vi "test.vi"() -> ()   [LabVIEW 2019]
uses:
  <vilib>/Platform/TimedLoop/XDataNode/timing_clust.ctl
  <vilib>/Platform/TimedLoop/XDataNode/nitl_modes.ctl
  <vilib>/Platform/TimedLoop/XDataNode/wakeup.ctl
  <vilib>/platform/TimedLoop/XDataNode/XDataNode.xnode
  KNRm_ReMi_OS6_436Motor.lvlibp
  <vilib>/Platform/TimedLoop/XDataNode/XDNodeRunTimeDep.lvlib
panel:
  out "Distance (cm)":cluster{"IR1":dbl, "IR2":dbl}
  in  "PulseRate&Dir P/S":dbl format="%#_13g"
  out "PulseCounter+/-":i32
  out "LimitBtn":bool
  in  "stop":bool
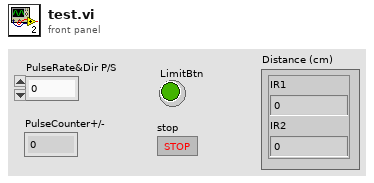
[diagram p1: front panel]
types:
  T1 = typedef "XDNodeRunTimeDep.lvlib/timing_clust.ctl" = cluster{"Expected End [f-1]":u64, "Actual End [f-1]":u64, "Finished Late? [f-1]":bool, "Expected End [i-1]":u64, "Actual End [i-1]":u64, "Finished Late? [i-1]":bool, "Expected Start [i]":u64, "Actual Start [i]":u64, "Expected Start [f]":u64, "Actual Start [f]":u64, "Source Name":string, "Structure Name":string, "Period":i64, "Deadline":i64, "Offset":i64, "Start":i64, "Priority":i32, "Timeout":i32, "Mode":T2, "Wakeup Reason":T3, "Error":errorcluster, "Source Type":string, "Secondary Source Type":string, "Global End Time":u64, "Global Start Time":u64, "Frame Duration":u64, "Iteration Duration":u64, "Assigned CPU":i32, "I/O Scan Engine Mode":u32}
  T2 = typedef "XDNodeRunTimeDep.lvlib/nitl_modes.ctl" = enum32{"No Change", "Process missed periods, maintain original phase", "Discard missed periods, maintain original phase", "Process missed periods, ignore original phase", "Discard missed periods, ignore original phase"}
  T3 = typedef "XDNodeRunTimeDep.lvlib/wakeup.ctl" = enum32{"Normal", "Aborted", "Asynchronous wakeup", "Timing source error", "Timed loop error", "Timeout"}
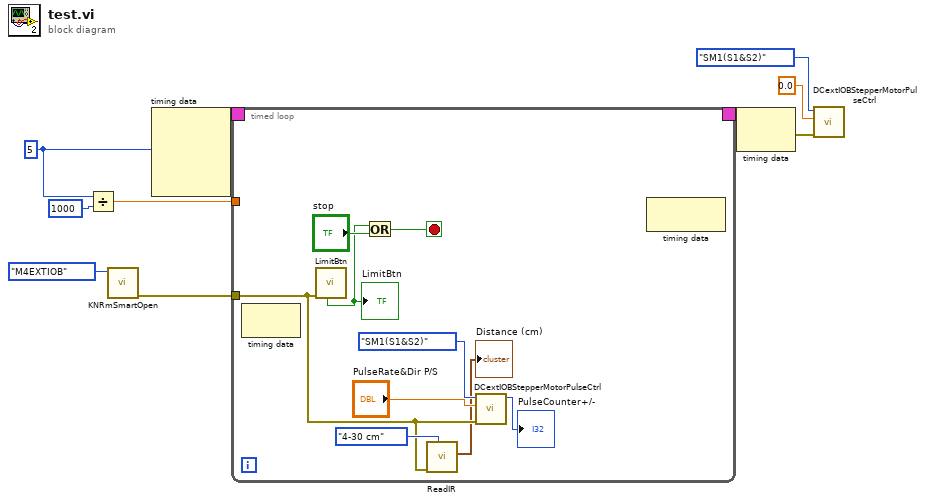
[diagram p0: block diagram]
diagram:
  w6 = i64 5 ("Period")
  n1 = Divide(x=w6, y=i64 1000) -> (x/y=w4:dbl)
  n2 = call "KNRmSmartOpen.vi"("INI FPGA MODE"=enum16{"Original", "M4EXTIOB"}."M4EXTIOB") -> ("error out"=w9:errorcluster)  [unwired: 7 in, 3 out]
  n3 = node-c288(w6) -> (w8:T1)  [unwired: 3 in]
  n4 = timed-loop {
    tunnel: w9 -> [w12]
    timing: w8 -> [_]
    timing-out: [_] -> w7
    tunnel: w4 -> [_]
    stop <- w17 stop-if-true
    n5 = node-c288() -> ()  [unwired: 1 in, 1 out]
    n6 = call "LimitBtn.vi"("error in"=w12) -> ("LimitBtn"=w16:bool)  [unwired: 9 in, 1 out]
    "LimitBtn" <- w16
    n7 = Or(x=w16, y="stop") -> (x .or. y?=w17:bool)
    n8 = call "ReadIR.vi"("type"=enum16{"10-80 cm", "4-30 cm"}."4-30 cm", "error in"=w12) -> ("Distance (cm)"=→"Distance (cm)":cluster{"IR1":dbl, "IR2":dbl})  [unwired: 7 in, 2 out]
    n9 = call "DCextIOBStepperMotorPulseCtrl.vi"("error in"=w12, "PulseRate&Dir P/S"="PulseRate&Dir P/S", "Port"=enum16{"SM1(S1&S2)", "SM2(S3&S4)", "SM3(S5&S6)"}."SM1(S1&S2)") -> ("PulseCounter+/-"=→"PulseCounter+/-":i32)  [unwired: 7 in, 1 out]
    n10 = node-c288() -> ()  [unwired: 1 in, 1 out]
  }
  n11 = node-c288(w7) -> (w1:errorcluster)
  n12 = call "DCextIOBStepperMotorPulseCtrl.vi"("error in"=w1, "PulseRate&Dir P/S"=0.0, "Port"=enum16{"SM1(S1&S2)", "SM2(S3&S4)", "SM3(S5&S6)"}."SM1(S1&S2)") -> ()  [unwired: 7 in, 2 out]
